vi "Save File.vi"(1 "Text in":string, 2 "Open Browser?":bool, 3 "file path (dialog if empty)":path) -> (0 "Text in":string)   [LabVIEW 2012]
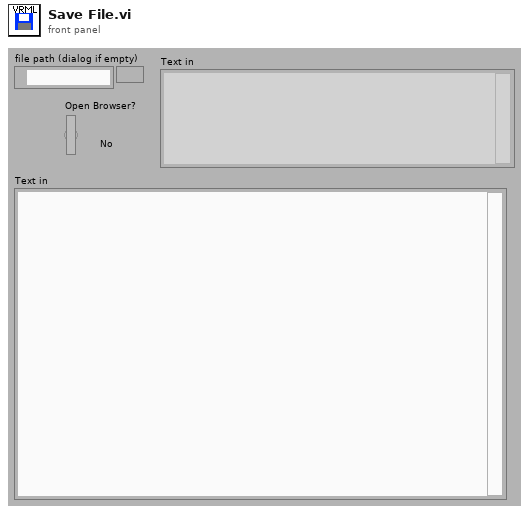
[diagram p1: front panel]
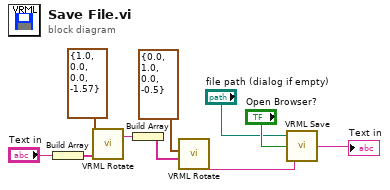
[diagram p0: block diagram]
diagram:
  n1 = Build Array("Text in") -> (w6:string[])
  n2 = call <userlib>:"VRML Rotate.vi"("Rotation"=cluster{"X":dbl, "Y":dbl, "Z":dbl, "theta":dbl} {"X"=1.0, "Y"=0.0, "Z"=0.0, "theta"=-1.57}, "Children"=w6) -> ("Text"=w4:string)  [unwired: 3 in, 1 out]
  n3 = Build Array(w4) -> (w3:string[])
  n4 = call <userlib>:"VRML Rotate.vi"("Rotation"=cluster{"X":dbl, "Y":dbl, "Z":dbl, "theta":dbl} {"X"=0.0, "Y"=1.0, "Z"=0.0, "theta"=-0.5}, "Children"=w3) -> ("Text"=w1:string)  [unwired: 3 in, 1 out]
  n5 = call <userlib>:"VRML Save.vi"("Text in"=w1, "Open Browser?"="Open Browser?", "file path (dialog if empty)"="file path (dialog if empty)") -> ("Text in"=→"Text in":string)
